vi "tkrsa6100 Binary to Sgl Float.vi"(10 "Digits of Precision":i32 max=12 step=1, 11 "Character String":string) -> (2 "Converted Numeric":dbl, 3 "Float String":string)   [LabVIEW 2020, in "Library Instrument & Equipement.lvlib" / "Library Spectrum Analyser.lvlib"]
doc: "This VI converts a 4 byte binary sample to a single precision floating point number.\n\nIt functions as follows:\n\nCharacter String is cast to a 32 bit unsigned interger and the bit order is reversed by the Swap Bytes and Swap Words functions.\n\nThe resulting 32 bit binary number is then cast to a single precision float and converted to a string for output to the calling function. Numeric control Digits of Precision (0) is passed to the float to string conversion function to make the number of digits of precision user-controllable."
uses:
  Library Spectrum Analyser.lvlib
panel:
  # "Little Endian String to Single Precision Float Converter"
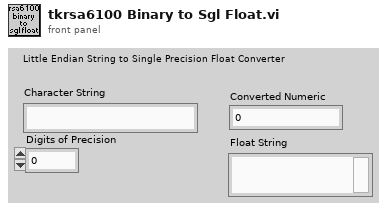
[diagram p1: front panel]
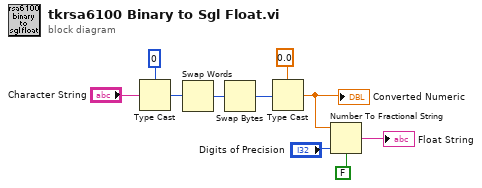
[diagram p0: block diagram]
diagram:
  n1 = Type Cast(type=u32 0, x="Character String") -> (*(type *) &x=w8:u32)
  n2 = Swap Words(1:w8) -> (0:w9:u32)
  n3 = Swap Bytes(anything=w9) -> (byte swapped=w10:u32)
  n4 = Type Cast(type=sgl 0.0, x=w10) -> (*(type *) &x=w7:sgl)
  "Converted Numeric" <- w7
  n5 = Number To Fractional String(use system decimal point (T)=FALSE, number=w7, precision (6)="Digits of Precision") -> (F-format string=→"Float String":string)  [unwired: 1 out]
